vi "DAQ@AnalogInWaveForm__Parameter.vi"(1 "ParamterIn":string) -> (0 "ParamterOut":string)   [LabVIEW 2020]
panel:
  in  "Second":string(combo)
  in  "WaveFrom":string(combo)
  in  "DAQName":string(combo)
  in  "Confirm":bool
  # "DAQ@AnalogInWaveForm $DAQ(,$Second,$WavefromName)"
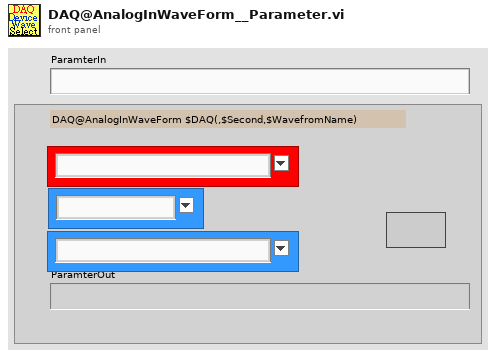
[diagram p1: front panel]
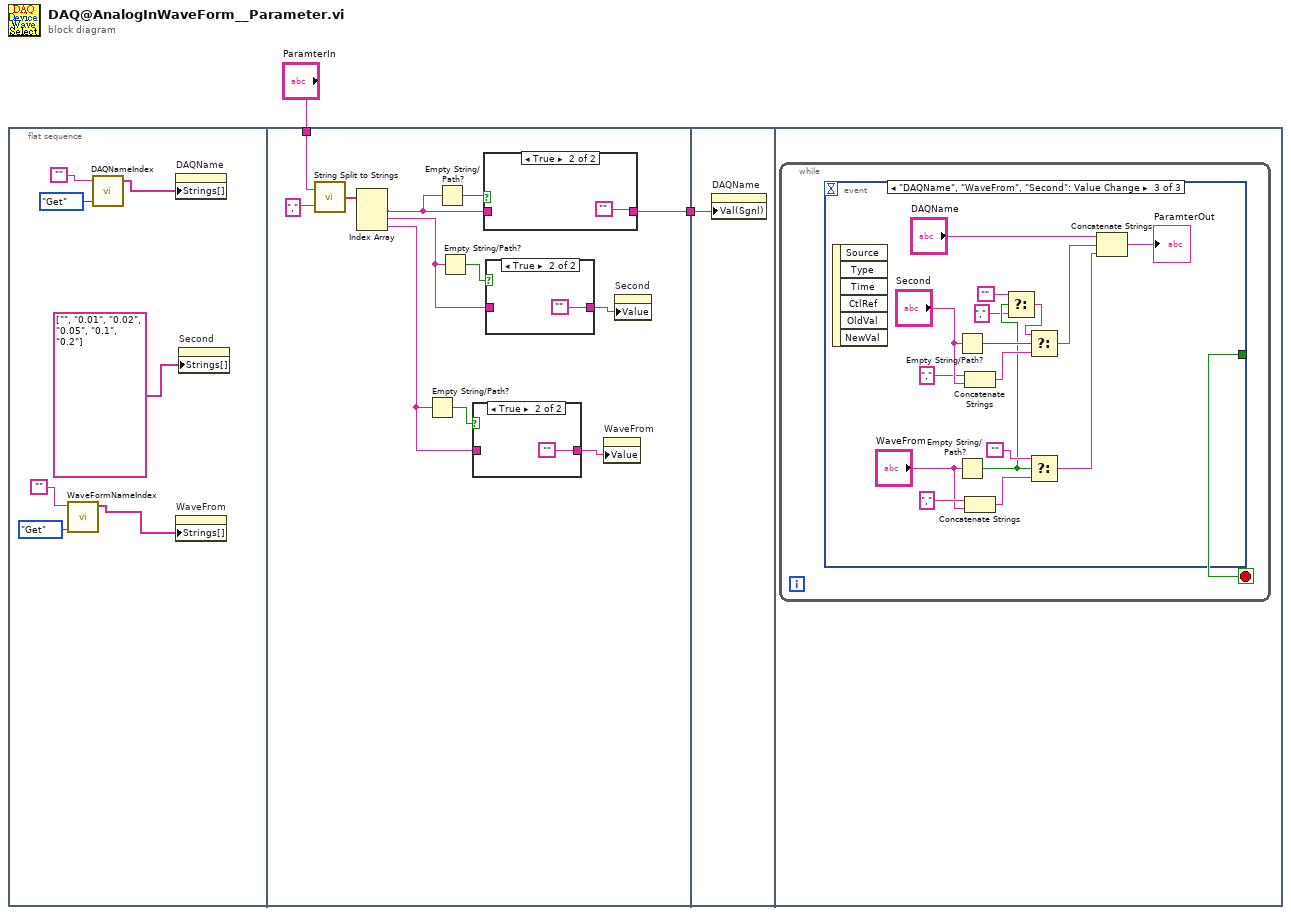
[diagram p0: block diagram]
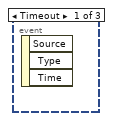
[diagram p5: hidden frame]
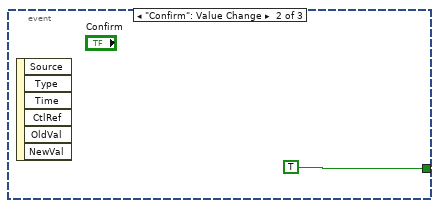
[diagram p6: hidden frame]
diagram:
  n1 = flat-sequence {
    tunnel: "ParamterIn" -> [w18]
    tunnel: [w14] -> w1
    tunnel: w1 -> [w28]
    frame #0 {
      n2 = call "WaveFormNameIndex.vi"("OP"=enum16{"Get", "Update", "Init", "GetSPS"}."Get", "WaveFormName"="") -> ("WaveFormNameList"=w4:string[])  [unwired: 6 in, 3 out]
      n3 = call "DAQNameIndex.vi"("OP"=enum16{"Get", "Update", "Init"}."Get", "DAQName"="") -> ("DAQList"=w7:string[])  [unwired: 1 in, 2 out]
      n4 = property on="DAQName" class="CmbBox"("Strings[]"=w7) -> ()  [unwired: 2 in, 2 out]
      n5 = property on="WaveFrom" class="CmbBox"("Strings[]"=w4) -> ()  [unwired: 2 in, 2 out]
      n6 = property on="Second" class="CmbBox"("Strings[]"=string[] ["", "0.01", "0.02", "0.05", "0.1", "0.2"] ("Strings []")) -> ()  [unwired: 2 in, 2 out]
    }
    frame #1 {
      n7 = call "String Split to Strings.vi"("search string/char (-)"=",", "String"=w18) -> ("Array"=w20:string[])
      n8 = Index Array(array=w20) -> (element #1=w17:string, element #2=w11:string, element #3=w13:string)  [unwired: 3 in]
      n9 = Empty String/Path?(string/path=w13) -> (empty?=w16:bool)
      n10 = Empty String/Path?(string/path=w17) -> (empty?=w21:bool)
      n11 = Empty String/Path?(string/path=w11) -> (empty?=w12:bool)
      n12 = case shown="True" w16 {
        tunnel: [w24 ""] -> w15
        tunnel: w13 -> [w24 _]
        frame False {
        }
        frame True {
        }
      }
      n13 = case shown="True" w21 {
        tunnel: w17 -> [w26 _]
        tunnel: [w26 ""] -> w14
        frame False {
        }
        frame True {
        }
      }
      n14 = case shown="True" w12 {
        tunnel: [w22 ""] -> w10
        tunnel: w11 -> [w22 _]
        frame False {
        }
        frame True {
        }
      }
      n15 = property on="WaveFrom" class="CmbBox"("Value"=w15) -> ()  [unwired: 2 in, 2 out]
      n16 = property on="Second" class="CmbBox"("Value"=w10) -> ()  [unwired: 2 in, 2 out]
    }
    frame #2 {
      n17 = property on="DAQName" class="CmbBox"("Val(Sgnl)"=w28) -> ()  [unwired: 2 in, 2 out]
    }
    frame #3 {
      n18 = while {
        stop <- w29 stop-if-true
        n19 = event shown="[2] \"DAQName\", \"WaveFrom\", \"Second\": Value Change" {
          selector: _ -> [_ _ _]
          dyn-events: _ -> [_ _ _]
          timeout: _ -> [_ _ _]
          tunnel: [_ TRUE _] -> w29
          event Timeout {
            n20 = event-data() -> ()  [unwired: 1 in, 3 out]
          }
          event "Confirm": Value Change {
            n21 = event-data() -> ()  [unwired: 1 in, 6 out]
          }
          event "DAQName", "WaveFrom", "Second": Value Change {
            n22 = event-data() -> ()  [unwired: 1 in, 6 out]
            n23 = Empty String/Path?(string/path="Second") -> (empty?=w37:bool)
            n24 = Empty String/Path?(string/path="WaveFrom") -> (empty?=w33:bool)
            n25 = Concatenate Strings("," ("string"), "Second") -> (w42:string)
            n26 = Concatenate Strings("," ("string"), "WaveFrom") -> (w40:string)
            n27 = Select(t="", s=w33, f=",") -> (s? t:f=w34:string)
            n28 = Select(t=w34, s=w37, f=w42) -> (s? t:f=w41:string)
            n29 = Select(t="", s=w33, f=w40) -> (s? t:f=w36:string)
            n30 = Concatenate Strings("DAQName", w41, w36) -> (→"ParamterOut":string)
          }
        }
      }
    }
  }
